vi "Write UUT.vi"(8 "error in":errorcluster, 10 "UUT":string, 11 "Chronometer in":refnum<class "Chronometer.lvclass">) -> (0 "error out":errorcluster, 3 "Chronometer out":refnum<class "Chronometer.lvclass">)   [LabVIEW 2023, in "Chronometer.lvlib" / "Chronometer.lvclass"]
uses:
  Chronometer.lvclass
  Chronometer.lvclass/Chronometer.ctl
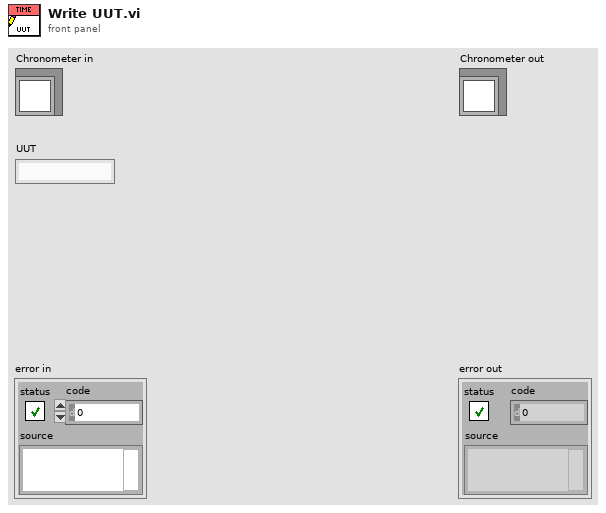
[diagram p1: front panel]
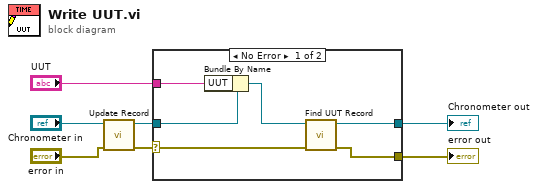
[diagram p0: block diagram]
diagram:
  n1 = call "Update Record.vi"("error in"="error in", "Chronometer in"="Chronometer in") -> ("error out"=w1:errorcluster, "Chronometer out"=w3:refnum<class "Chronometer.lvclass">)  [unwired: 8 in]
  n2 = case shown="No Error" w1 {
    selector: w1 -> [w8 w14]
    tunnel: [w10 w14] -> w7
    tunnel: [w11 w15] -> w6
    tunnel: w3 -> [w9 w15]
    tunnel: "UUT" -> [w13 _]
    frame No Error {
      n3 = Bundle By Name(cluster=w9, "UUT"=w13) -> (w12:refnum<class "Chronometer.lvclass">)
      n4 = call "Find UUT Record.vi"("error in"=w8, "Chronometer in"=w12) -> ("error out"=w10:errorcluster, "Chronometer out"=w11:refnum<class "Chronometer.lvclass">)  [unwired: 8 in]
    }
    frame Error {
    }
  }
  "error out" <- w7
  "Chronometer out" <- w6
